vi "Inscription.vi"() -> ()   [LabVIEW 2015]
uses:
  <vilib>/httpClient/LabVIEWHTTPClient.lvlib
panel:
  out "Tab Control 6":enum32{"Page 1", "Page 2"}(tab)
  out "Tab Control 5":enum32{"Page 1", "Page 2"}(tab)
  out "Tab Control 4":enum32{"Page 1", "Page 2"}(tab)
  out "Tab Control 3":enum32{"Page 1", "Page 2"}(tab)
  out "Tab Control 2":enum32{"Page 1", "Page 2"}(tab)
  in  "pwd":string
  in  "login":string
  in  "mail":string
  in  "gsm":string
  in  "OK Button 4":bool
  in  "OK Button 2":bool
  out "Tab Control":enum32{"Page 1", "Page 2"}(tab)
  in  "nom":string
  in  "cin":string
  # "Entrer Cin"
  # "Entrer Nom"
  # "Entrer GSM"
  # "Entrer Email"
  # "Entrer Login"
  # "Entrer Mot de passe"
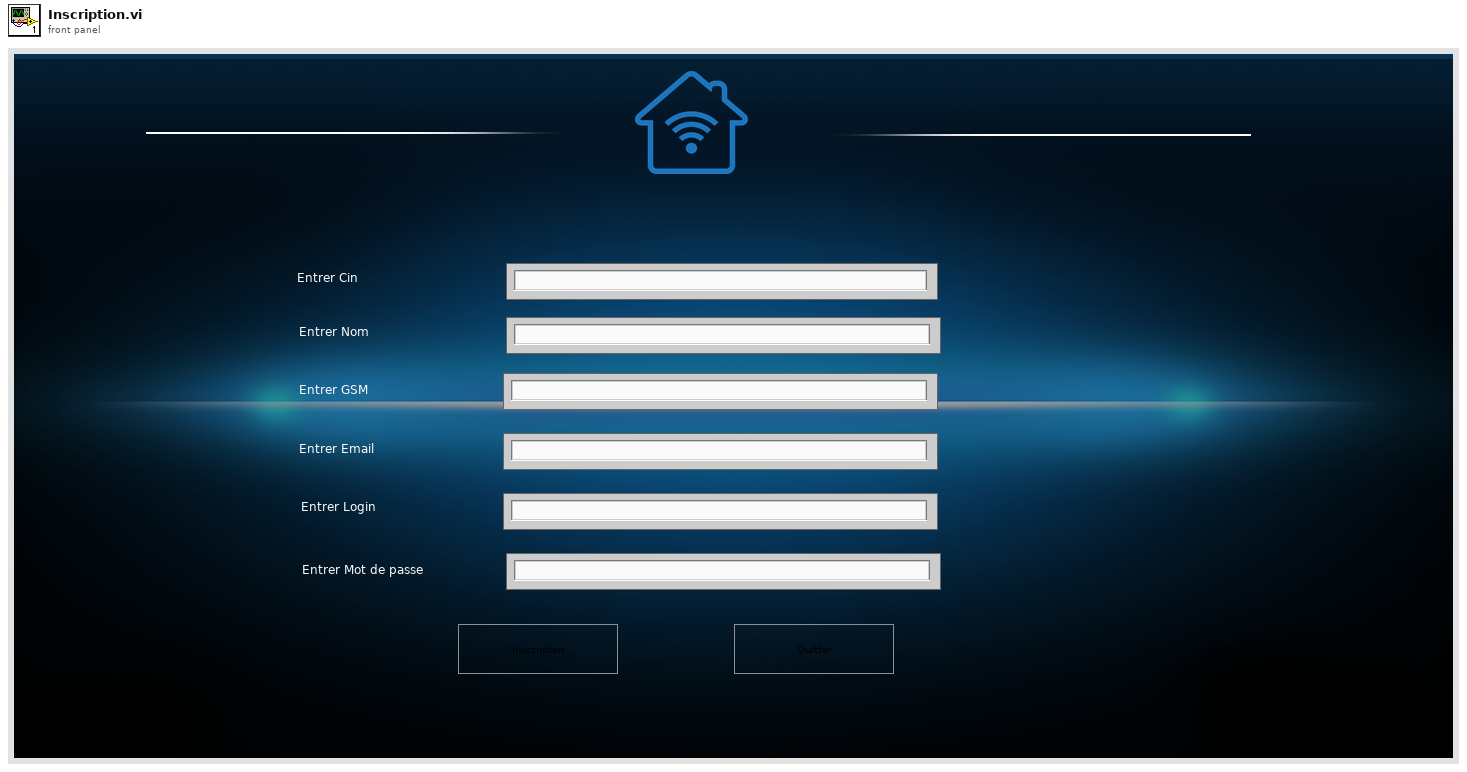
[diagram p1: front panel]
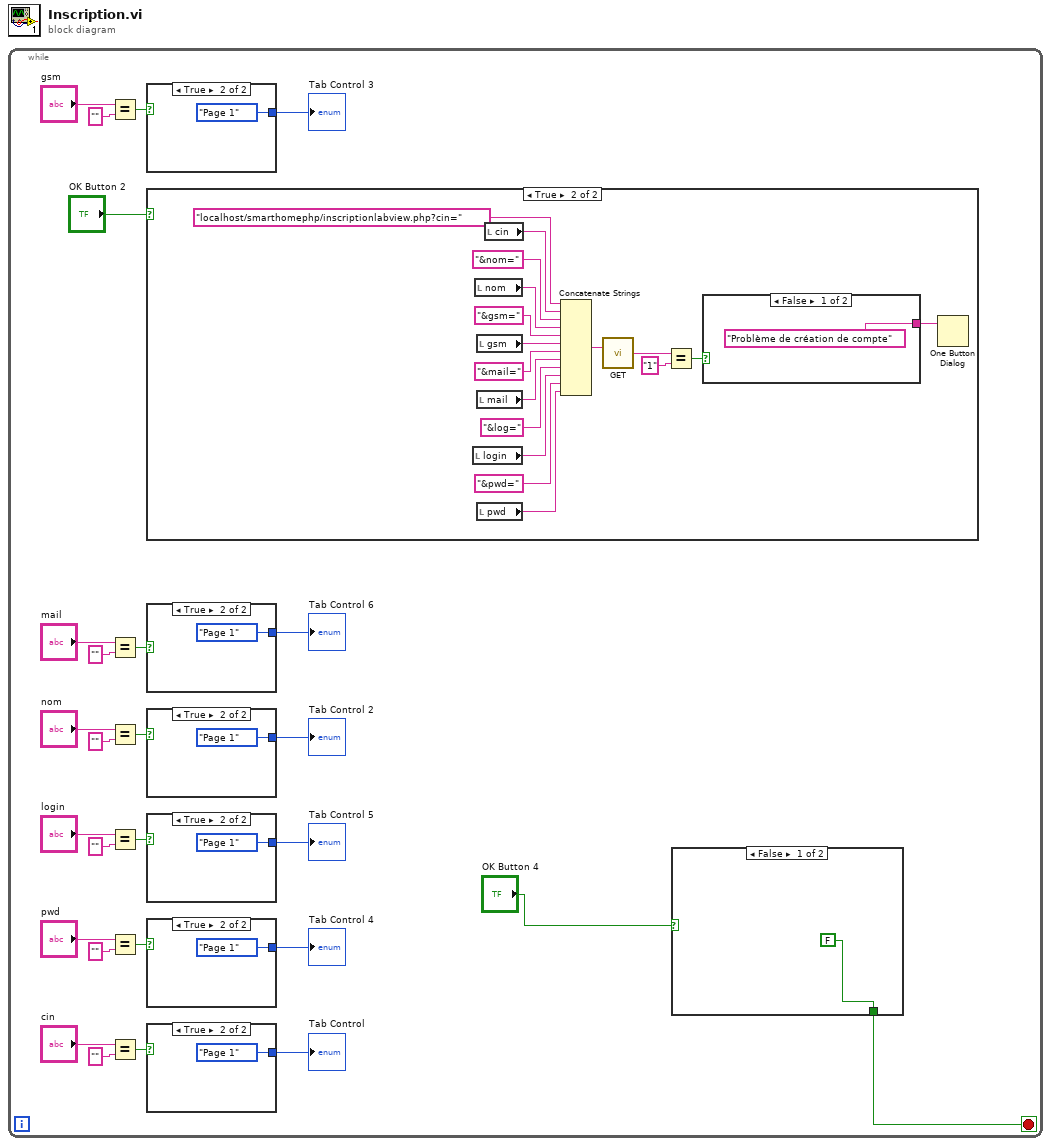
[diagram p0: block diagram]
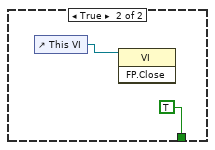
[diagram p2: hidden frame]
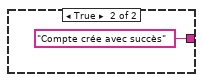
[diagram p4: hidden frame]
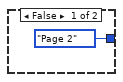
[diagram p5: hidden frame]
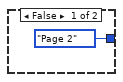
[diagram p6: hidden frame]
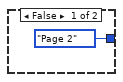
[diagram p7: hidden frame]
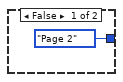
[diagram p8: hidden frame]
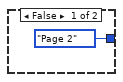
[diagram p9: hidden frame]
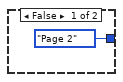
[diagram p10: hidden frame]
diagram:
  n1 = while {
    stop <- w2 stop-if-true
    n2 = Equal?(x="gsm", y="") -> (x = y?=w5:bool)
    n3 = Equal?(x="mail", y="") -> (x = y?=w9:bool)
    n4 = Equal?(x="nom", y="") -> (x = y?=w22:bool)
    n5 = Equal?(x="login", y="") -> (x = y?=w12:bool)
    n6 = Equal?(x="pwd", y="") -> (x = y?=w14:bool)
    n7 = Equal?(x="cin", y="") -> (x = y?=w23:bool)
    n8 = case shown="True" w5 {
      tunnel: [enum32{"Page 1", "Page 2"}."Page 2" ("Tab Control") enum32{"Page 1", "Page 2"}."Page 1" ("Tab Control")] -> w4
      frame False {
      }
      frame True {
      }
    }
    "Tab Control 3" <- w4
    n9 = case shown="True" "OK Button 2" {
      frame False {
      }
      frame True {
        n10 = local read "login"() -> (w38:string)
        n11 = local read "nom"() -> (w44:string)
        n12 = local read "gsm"() -> (w42:string)
        n13 = local read "mail"() -> (w40:string)
        n14 = local read "pwd"() -> (w36:string)
        n15 = local read "cin"() -> (w46:string)
        n16 = Concatenate Strings("localhost/smarthomephp/inscriptionlabview.php?cin=", w46, "&nom=", w44, "&gsm=", w42, "&mail=", w40, "&log=", w38, "&pwd=", w36) -> (w35:string)
        n17 = call <vilib>:"GET.vi"("url"=w35) -> ("body"=w34:string)  [unwired: 11 in, 3 out]
        n18 = Equal?(x=w34, y="1") -> (x = y?=w32:bool)
        n19 = case shown="False" w32 {
          tunnel: ["Problème de création de compte" "Compte crée avec succès"] -> w31
          frame False {
          }
          frame True {
          }
        }
        n20 = One Button Dialog(message=w31) -> ()  [unwired: 1 in, 1 out]
      }
    }
    n21 = case shown="True" w9 {
      tunnel: [enum32{"Page 1", "Page 2"}."Page 2" ("Tab Control") enum32{"Page 1", "Page 2"}."Page 1" ("Tab Control")] -> w8
      frame False {
      }
      frame True {
      }
    }
    "Tab Control 6" <- w8
    n22 = case shown="True" w22 {
      tunnel: [enum32{"Page 1", "Page 2"}."Page 2" ("Tab Control") enum32{"Page 1", "Page 2"}."Page 1" ("Tab Control")] -> w20
      frame False {
      }
      frame True {
      }
    }
    "Tab Control 2" <- w20
    n23 = case shown="True" w12 {
      tunnel: [enum32{"Page 1", "Page 2"}."Page 2" ("Tab Control") enum32{"Page 1", "Page 2"}."Page 1" ("Tab Control")] -> w11
      frame False {
      }
      frame True {
      }
    }
    "Tab Control 5" <- w11
    n24 = case shown="True" w14 {
      tunnel: [enum32{"Page 1", "Page 2"}."Page 2" ("Tab Control") enum32{"Page 1", "Page 2"}."Page 1" ("Tab Control")] -> w7
      frame False {
      }
      frame True {
      }
    }
    "Tab Control 4" <- w7
    n25 = case shown="True" w23 {
      tunnel: [enum32{"Page 1", "Page 2"}."Page 2" ("Tab Control") enum32{"Page 1", "Page 2"}."Page 1" ("Tab Control")] -> w21
      frame False {
      }
      frame True {
      }
    }
    "Tab Control" <- w21
    n26 = case shown="False" "OK Button 4" {
      tunnel: [FALSE TRUE] -> w2
      frame False {
      }
      frame True {
        n27 = control-ref of="This VI"() -> (w30:refnum<vi>)
        n28 = invoke class="VI" method="FP.Close"(reference=w30) -> ()  [unwired: 2 in, 3 out]
      }
    }
  }
